vi "Device_Close.vi"(8 "Device Handler Pointer":i64[](array[numeric]), 9 "Selected Count":i32, 10 "queue out":refnum<queue>, 11 "refnum out":refnum<file>) -> ()   [LabVIEW 2026]
uses:
  x64/Release/CanSharkApi_Dll1.dll
panel:
  in  "datalog":bool
  out "return type":i32
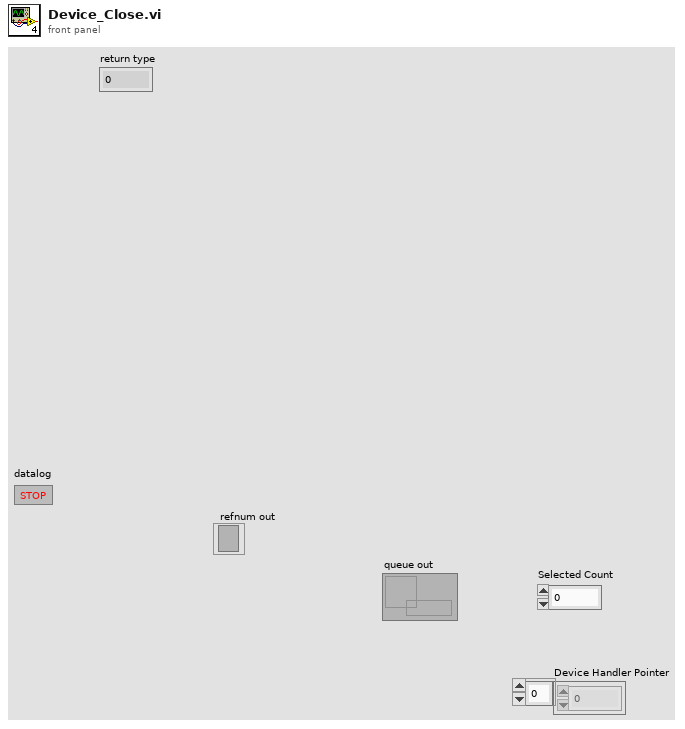
[diagram p1: front panel]
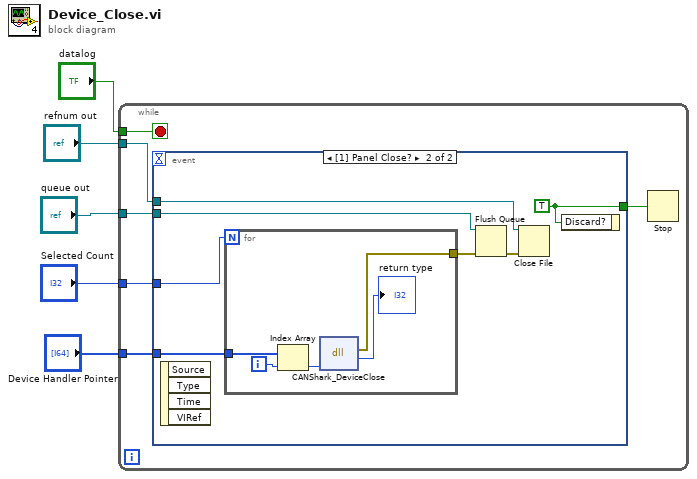
[diagram p0: block diagram]
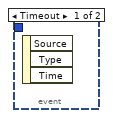
[diagram p2: hidden frame]
diagram:
  n1 = while {
    tunnel: "Device Handler Pointer" -> [w11]
    tunnel: "Selected Count" -> [w10]
    tunnel: "refnum out" -> [w9]
    tunnel: "datalog" -> [w8]
    tunnel: "queue out" -> [w6]
    stop <- w8 stop-if-true
    n2 = event shown="[1] Panel Close?" {
      selector: _ -> [_ _]
      dyn-events: _ -> [_ _]
      timeout: _ -> [_ _]
      tunnel: w11 -> [_ w17]
      tunnel: w10 -> [_ w18]
      tunnel: w9 -> [_ w13]
      tunnel: [_ w16] -> w7
      tunnel: w6 -> [_ w14]
      event Timeout {
        n3 = event-data() -> ()  [unwired: 1 in, 3 out]
      }
      event Panel Close? {
        w16 = TRUE
        n4 = event-data() -> ()  [unwired: 1 in, 4 out]
        n5 = for {
          N: w18 -> [_]
          tunnel: w17 -> [w20]
          tunnel: [w19] -> w15
          i -> [w21]
          n6 = Index Array(array=w20, index=w21) -> (element=w23:i64)
          n7 = dll-call lib="C:/Users/TECQNIO/Documents/CANSHARK LABVIEW API PACKAGE/x64/Release/CanSharkApi_Dll1.dll" fn="CANShark_DeviceClose"("Device"=w23) -> (error out=w19:errorcluster, "return type"=→"return type":i32)  [unwired: 4 in, 1 out]
        }
        n8 = Flush Queue(queue=w14, error in (no error)=w15) -> (error out=w12:errorcluster)  [unwired: 2 out]
        n9 = Close File(refnum=w13, error in=w12) -> ()  [unwired: 2 out]
        n10 = event-data("Discard?"=w16) -> ()  [unwired: 1 in, 1 out]
      }
    }
    n11 = Stop(stop? (T)=w7) -> ()
  }
